vi "last part of path.vi"(11 "String":string) -> (0 "Last Part":string)   [LabVIEW 2011]
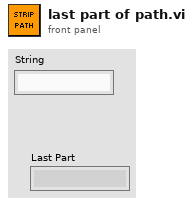
[diagram p1: front panel]
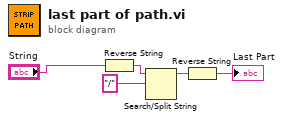
[diagram p0: block diagram]
diagram:
  n1 = Reverse String(1:"String") -> (0:w5:string)
  n2 = Search/Split String(string=w5, search string/char (-)="/") -> (substring before match=w4:string)  [unwired: 1 in, 2 out]
  n3 = Reverse String(1:w4) -> (0:→"Last Part":string)
